vi "Hangup Auswertung.vi"() -> (0 "Bestanden":bool, 2 "Ergebnis ppmC1 2":sgl, 3 "Ergebnis ppmC3":sgl)   [LabVIEW 2020, in "Hangup Check.lvlib"]
uses:
  Hangup Check.lvlib
  AktionFGV Hangup.ctl
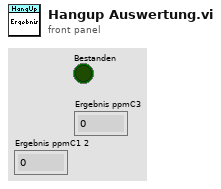
[diagram p1: front panel]
types:
  T1 = typedef "Hangup Check.lvlib/AktionFGV Hangup.ctl" = enum16{"lesen", "Hangup Settings", "Protokoll", "Pfad", "laden", "speichern"}
  T2 = typedef "Hangup Check.lvlib/HangupSettings.ctl" = cluster{"Kalibriergas":T3, "Aufschaltpunkt":T3, "Spangas Aufschaltzeit:":sgl, "Nullgas Aufschaltzeit:":sgl, "Datenerfassungszeit:":sgl, "Grenzwert manuell:":sgl, "Grenzwert:":sgl, "Grenze":T3, "Messbereich":T3, "Spankonzentration [ppm]":sgl, "Grenzwert: C1":sgl}
  T3 = typedef "Auswahlfeld.ctl" = u16
  T4 = typedef "Hangup Check.lvlib/Protokoll.ctl" = cluster{"FID Mittelwert 0":sgl, "FID Mittelwert E":sgl, "Messgasdruck Amium":sgl, "Startzeit":timestamp, "Endzeit":timestamp, "Bestanden?":bool}
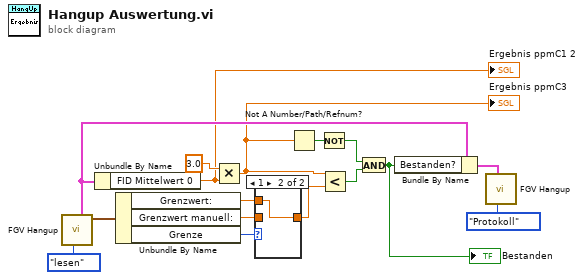
[diagram p0: block diagram]
diagram:
  n1 = call "FGV Hangup.vi"("Aktion"=AktionFGV_Hangup."lesen") -> ("Hangup Settings"=w4:T2, "Protokoll"=w13:T4)  [unwired: 6 in, 3 out]
  n2 = Unbundle By Name(w13) -> ("FID Mittelwert 0"=w1:sgl)
  "Ergebnis ppmC1 2" <- w1
  n3 = Unbundle By Name(w4) -> ("Grenzwert:"=w8:sgl, "Grenzwert manuell:"=w9:sgl, "Grenze"=w7:T3)
  n4 = Multiply(x=sgl 3.0, y=w1) -> (x*y=w6:sgl)
  "Ergebnis ppmC3" <- w6
  n5 = case shown="1" w7 {
    tunnel: w8 -> [_ w18]
    tunnel: w9 -> [w17 _]
    tunnel: [w17 w18] -> w10
    frame 0, Default {
    }
    frame 1 {
    }
  }
  n6 = Not A Number/Path/Refnum?(number/path/refnum=w6) -> (NaN/Path/Refnum?=w11:bool)
  n7 = Not(x=w11) -> (.not. x?=w16:bool)
  n8 = Less?(x=w6, y=w10) -> (x < y?=w12:bool)
  n9 = And(x=w16, y=w12) -> (x .and. y?=w2:bool)
  "Bestanden" <- w2
  n10 = Bundle By Name(cluster=w13, "Bestanden?"=w2) -> (w15:T4)
  n11 = call "FGV Hangup.vi"("Aktion"=AktionFGV_Hangup."Protokoll", "Protokoll"=w15) -> ()  [unwired: 5 in, 5 out]
